vi "開啟圖片(1D).vi"(8 "error In":errorcluster, 10 "影像數量":i32=1, 11 "Image Name":string="Source") -> (0 "error out":errorcluster, 1 "ImageOutNameArray":string[](array[string]), 2 "ImagePathNumber":i32, 3 "Image1DArray":T1[](array[typedef]), 5 "ImagePath":path[](array[path]))   [LabVIEW 2015]
uses:
  <vilib>/vision/Image Controls.llb/IMAQ Image.ctl
  Image action.ctl
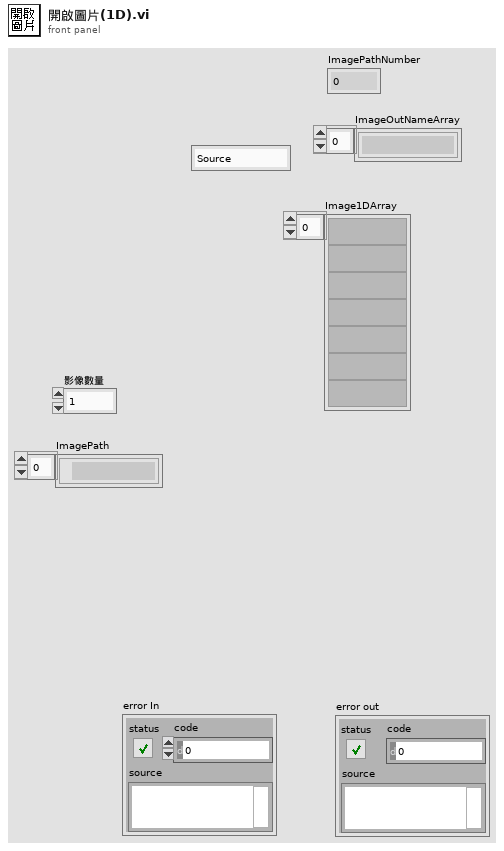
[diagram p1: front panel]
types:
  T1 = typedef "IMAQ Image.ctl" = refnum<image>
  T2 = typedef "Image action.ctl" = enum16{"初始化", "創造記憶體", "寫入圖片", "讀取圖片", "刪除圖片", "等待"}
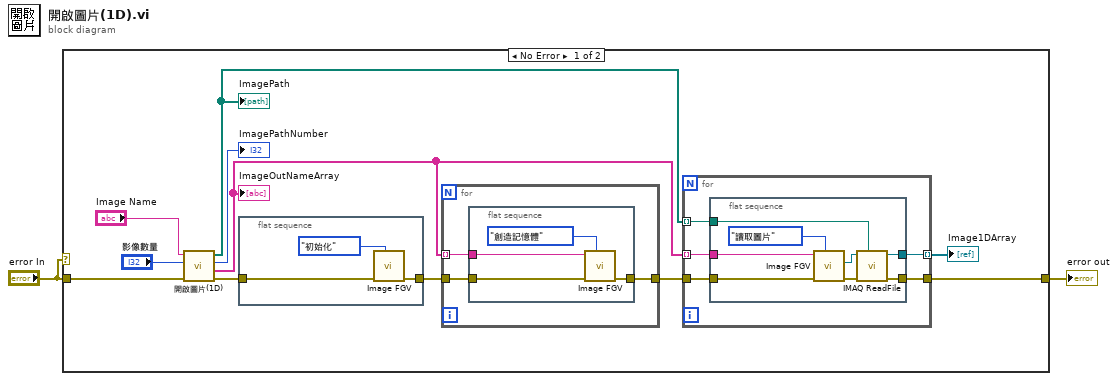
[diagram p0: block diagram]
diagram:
  n1 = case shown="No Error" "error In" {
    tunnel: [w11 w37] -> w2
    tunnel: "error In" -> [w12 w37]
    frame No Error {
      n2 = call "開啟圖片(1D).vi"("error In"=w12, "影像數量"="影像數量", "Image Name"="Image Name") -> ("error out"=w5:errorcluster, "ImageOutNameArray"=w6:string[], "ImagePathNumber"=→"ImagePathNumber":i32, "ImagePath"=w7:path[])  [unwired: 5 in]
      "ImageOutNameArray" <- w6
      "ImagePath" <- w7
      n3 = flat-sequence {
        tunnel: [w35] -> w9
        tunnel: w5 -> [w34]
        frame #0 {
          n4 = call "Image FGV.vi"("Image action"=Image_action."初始化", "error in (no error)"=w34) -> ("error out"=w35:errorcluster)  [unwired: 8 in, 1 out]
        }
      }
      n5 = for {
        tunnel: w9 -> [w29]
        tunnel: w6 -> [w28] mode=indexing
        tunnel: [w27] -> w8
        n6 = flat-sequence {
          tunnel: w29 -> [w32]
          tunnel: w28 -> [w31]
          tunnel: [w30] -> w27
          frame #0 {
            n7 = call "Image FGV.vi"("Image action"=Image_action."創造記憶體", "error in (no error)"=w32, "圖片名稱"=w31) -> ("error out"=w30:errorcluster)  [unwired: 7 in, 1 out]
          }
        }
      }
      n8 = for {
        tunnel: w8 -> [w18]
        tunnel: w6 -> [w17] mode=indexing
        tunnel: w7 -> [w16] mode=indexing
        tunnel: [w15] -> w13 mode=indexing
        tunnel: [w14] -> w11
        n9 = flat-sequence {
          tunnel: w18 -> [w25]
          tunnel: w17 -> [w24]
          tunnel: w16 -> [w23]
          tunnel: [w21] -> w15
          tunnel: [w19] -> w14
          frame #0 {
            n10 = call "Image FGV.vi"("Image action"=Image_action."讀取圖片", "error in (no error)"=w25, "圖片名稱"=w24) -> ("error out"=w20:errorcluster, "Image Out"=w22:T1)  [unwired: 7 in]
            n11 = call "IMAQ ReadFile"("File Path"=w23, "error in (no error)"=w20, "Image"=w22) -> ("error out"=w19:errorcluster, "Image Out"=w21:T1)  [unwired: 4 in, 3 out]
          }
        }
      }
      "Image1DArray" <- w13
    }
    frame Error {
    }
  }
  "error out" <- w2
